vi "RLY_Select.vi"(2 "error in":errorcluster, 3 "RLY":T1) -> (0 "error out":errorcluster, 1 "hex string":string)   [LabVIEW 2019]
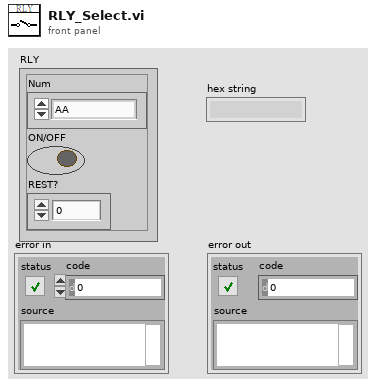
[diagram p1: front panel]
types:
  T1 = cluster{"Num":enum16{"AA", "01", "02", "03", "04", "05", "06", "07", "08", "09", "10", "11", "12", "13", "14", "15", "16", "17", "18", "19", "20", "21", "22", "23", "24"}, "ON/OFF":bool, "REST?":u16}
  T2 = enum16{"AA", "01", "02", "03", "04", "05", "06", "07", "08", "09", "10", "11", "12", "13", "14", "15", "16", "17", "18", "19", "20", "21", "22", "23", "24"}
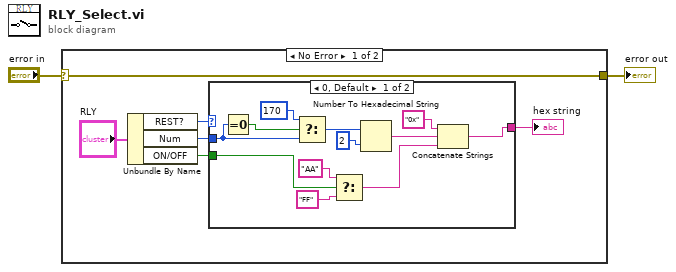
[diagram p0: block diagram]
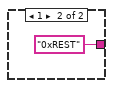
[diagram p2: hidden frame]
diagram:
  n1 = case shown="No Error" "error in" {
    selector: "error in" -> [w7 w22]
    tunnel: [w7 w22] -> w1
    frame No Error {
      n2 = Unbundle By Name("RLY") -> ("REST?"=w5:u16, "Num"=w3:T2, "ON/OFF"=w4:bool)
      n3 = case shown="0, Default" w5 {
        tunnel: [w17 "0xREST"] -> w8
        tunnel: w4 -> [w10 _]
        tunnel: w3 -> [w9 _]
        frame 0, Default {
          n4 = Equal To 0?(x=w9) -> (x = 0?=w13:bool)
          n5 = Select(t=170 ("number"), s=w13, f=w9) -> (s? t:f=w11:i32)
          n6 = Select(t="AA", s=w10, f="FF") -> (s? t:f=w14:string)
          n7 = Number To Hexadecimal String(1:i16 2 ("width (-)"), 2:w11) -> (0:w18:string)
          n8 = Concatenate Strings("0x" ("string"), w18, w14) -> (w17:string)
        }
        frame 1 {
        }
      }
      "hex string" <- w8
    }
    frame Error {
    }
  }
  "error out" <- w1
